vi "pco.labview_LightSheet_Example.vi"() -> ()   [LabVIEW 2019]
uses:
  pco.sdk/CameraAccess/CameraAccess.lvlib
  pco.sdk/Structures/Structures.lvlib
  pco.recorder/Recorder.lvlib
  pco.sdk/RecordingControl/RecordingControl.lvlib
  pco.sdk/TimingControl/TimingControl.lvlib
  pco.sdk/GeneralCameraControl/GeneralCameraControl.lvlib
  pco.sdk/SpecialCommandsEdge/SpecialCommandsEdge.lvlib
panel:
  in  "dwExposureLines":u32=100
  in  "wTimeBase":u16(ring)=1 items=["ns", "us", "ms"]
  in  "dwLineTime":u32=50
  out "Recorded Images":u32
  out "Image":u16[][](graph)
  in  "Quit":bool
  in  "roiY1":u16=2 min=2 step=1
  in  "roiX1":u16=2 min=2 step=1
  in  "roiY0":u16=1 min=1 step=1
  in  "roiX0":u16=1 min=1 step=1
  out "Image Height":u16
  out "Image Width":u16
  in  "Image Index":u32 max=9
  in  "dwImgCount":u32=10 caption="Required Number of Images" max=4023
  out "Error":errorcluster {"code" format="%x"}
  # "This example is similar to the simple example, but uses get/set line timeing for controlling the exposure.\nExposureTime = LineTime * ExposureLines\nBeside of the line timing part, a simple recording of an image sequence and the image access afterwards is done.\nIt is a good starting point for writing own applications, especially  for light sheet application development.\nBut it will not be fail save, i.e. doesnt react on errors, just handles them forward to the end\n\nUsage:\nSelect your required image count and the required line tiime + number of exposure lines before you start the program.\nOnce started, the camera will be opened, the recorder will be created, initialized and images will be recorded automatically.\nWhen acquisition has finished you can address the images and set a certain roi \nTo finish the program click on quit application, this will force free and delete of the recorder and a close camera"
  # "pco.labview"
  # "Camera Setup"
  # "Recording Control"
  # "Parameters for image readout"
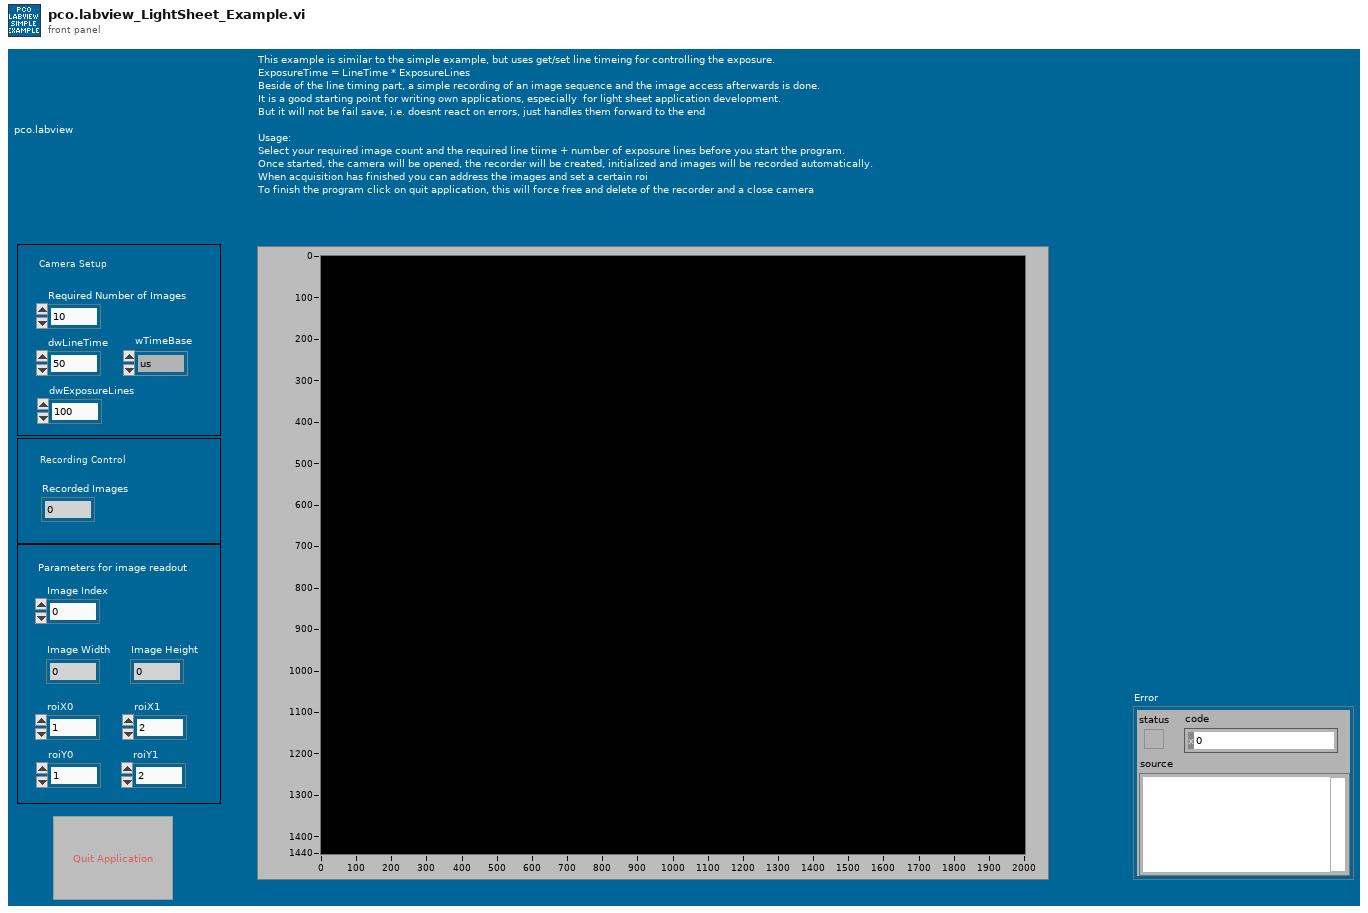
[diagram p1: front panel]
types:
  T1 = enum8{"Enabled", "Disabled", "Disabled and Grayed Out"}
  T2 = cluster{"wInterfaceType":u16, "wCameraNumber":u16, "wCameraNumAtInterface":u16, "wOpenFlags":u16[], "dwOpenFlags":u32[], "wOpenPtr":u64[]}
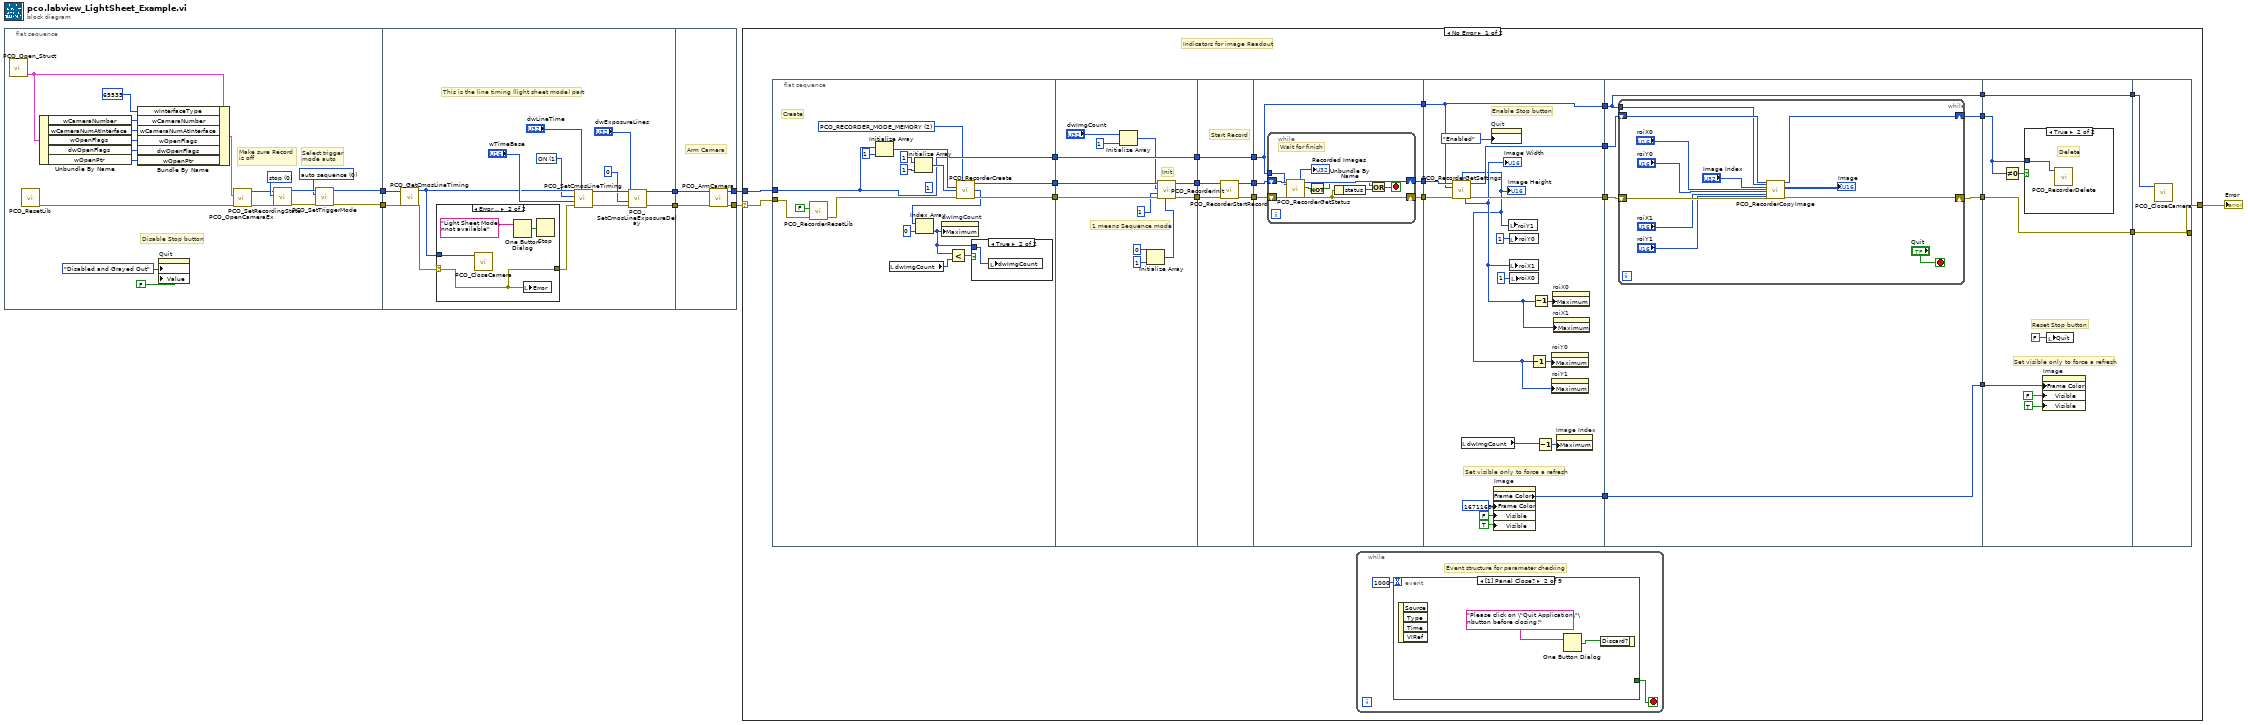
[diagram p0: block diagram]
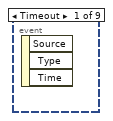
[diagram p3: hidden frame]
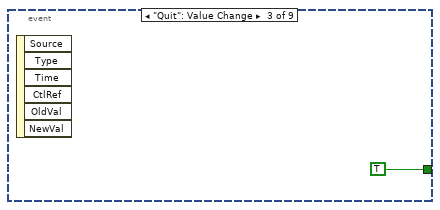
[diagram p4: hidden frame]
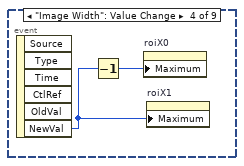
[diagram p5: hidden frame]
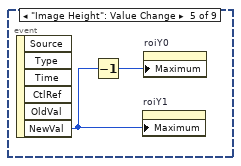
[diagram p6: hidden frame]
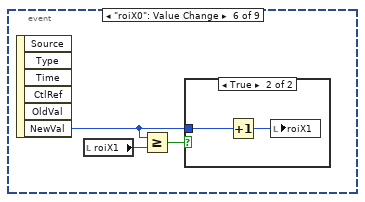
[diagram p7: hidden frame]
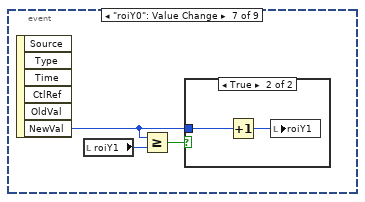
[diagram p9: hidden frame]
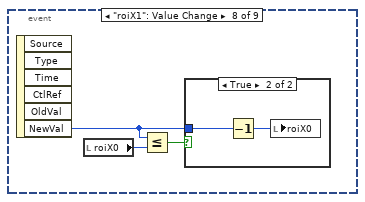
[diagram p11: hidden frame]
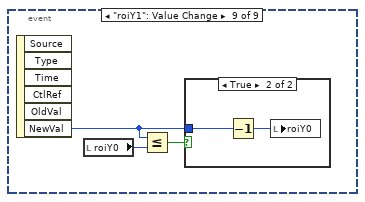
[diagram p13: hidden frame]
diagram:
  n1 = flat-sequence {
    tunnel: [w9] -> w4
    tunnel: [w8] -> w3
    tunnel: w4 -> [w39]
    tunnel: w3 -> [w40]
    tunnel: [w30] -> w2
    tunnel: [w29] -> w1
    tunnel: [w48] -> w5
    tunnel: [w49] -> w7
    tunnel: w2 -> [w47]
    tunnel: w1 -> [w46]
    frame #0 {
      w10 = u16 0 items=["auto sequence"=0, "software trigger"=1, "external exposure start & software trigger"=2, "external exposure control"=3, "external synchronized"=4, "fast external exposure control"=5, "external CDS control"=6, "slow external exposure control"=7, "external synchronized HDSDI"=258] ("wTriggerMode")
      w15 = u16 0 items=["stop", "run"] ("wRecState")
      # "Select trigger\nmode auto"
      # "Make sure Record \nis off"
      # "Disable Stop button"
      n2 = call "PCO_Open_Struct.vi"() -> ("PCO_Open_Struct"=w22:T2)  [unwired: 4 in, 4 out]
      n3 = call "PCO_ResetLib.vi"() -> ("error out"=w26:errorcluster)  [unwired: 10 in, 1 out]
      n4 = Unbundle By Name(w22) -> ("wCameraNumber"=w21:u16, "wCameraNumAtInterface"=w20:u16, "wOpenFlags"=w19:u16[], "dwOpenFlags"=w18:u32[], "wOpenPtr"=w17:u64[])
      n5 = Bundle By Name(cluster=w22, "wInterfaceType"=u16 65535, "wCameraNumber"=w21, "wCameraNumAtInterface"=w20, "wOpenFlags"=w19, "dwOpenFlags"=w18, "wOpenPtr"=w17) -> (w16:T2)
      n6 = property on="Quit" class="Bool (strict)"("DisabledEnum"=T1."Disabled and Grayed Out" ("Disabled"), "Value"=FALSE ("Stop")) -> ()  [unwired: 2 in, 2 out]
      n7 = call "PCO_OpenCameraEx.vi"("error in (no error)"=w26, "strOpenStruct"=w16) -> ("error out"=w14:errorcluster, "ph out"=w13:u64)  [unwired: 7 in, 1 out]
      n8 = call "PCO_SetRecordingState.vi"("error in (no error)"=w14, "wRecState"=w15, "ph"=w13) -> ("error out"=w11:errorcluster, "ph out"=w12:u64)  [unwired: 6 in, 1 out]
      n9 = call "PCO_SetTriggerMode.vi"("error in (no error)"=w11, "wTriggerMode"=w10, "ph"=w12) -> ("error out"=w8:errorcluster, "ph out"=w9:u64)  [unwired: 6 in, 1 out]
    }
    frame #1 {
      w27 = u16 1 items=["OFF", "ON"] ("wParameter")
      # "This is the line timing (light sheet mode) part"
      n10 = call "PCO_GetCmosLineTiming.vi"("ph"=w39, "error in (no error)"=w40) -> ("ph out"=w28:u64, "error out"=w38:errorcluster)  [unwired: 10 in, 6 out]
      n11 = case shown="Error .." w38 {
        selector: w38 -> [w41 w42]
        tunnel: [w41 w42] -> w37
        tunnel: w28 -> [_ w43]
        frame No Error {
        }
        frame Error {
          n12 = call "PCO_CloseCamera.vi"("ph"=w43) -> ()  [unwired: 9 in, 2 out]
          n13 = One Button Dialog(message="Light Sheet Mode\nnot available") -> (true=w44:bool)  [unwired: 1 in]
          n14 = local write "Error"(w42) -> ()
          n15 = Stop(stop? (T)=w44) -> ()
        }
      }
      n16 = call "PCO_SetCmosLineTiming.vi"("dwLineTime"="dwLineTime", "error in (no error)"=w37, "wTimeBase"="wTimeBase", "wParameter"=w27, "ph"=w28) -> ("error out"=w33:errorcluster, "ph out"=w34:u64)  [unwired: 4 in, 1 out]
      n17 = call "PCO_SetCmosLineExposureDelay.vi"("error in (no error)"=w33, "dwDelayLines"=u32 0, "dwExposureLines"="dwExposureLines", "ph"=w34) -> ("error out"=w29:errorcluster, "ph out"=w30:u64)  [unwired: 5 in, 1 out]
    }
    frame #2 {
      # "Arm Camera"
      n18 = call "PCO_ArmCamera.vi"("error in (no error)"=w46, "ph"=w47) -> ("error out"=w48:errorcluster, "ph out"=w49:u64)  [unwired: 7 in, 1 out]
    }
  }
  n19 = case shown="No Error" w5 {
    selector: w5 -> [w54 w201]
    tunnel: [w50 w201] -> w6
    tunnel: w7 -> [w74 _]
    frame No Error {
      # "Indicators for image Readout"
      n20 = flat-sequence {
        tunnel: w74 -> [w114]
        tunnel: w54 -> [w111]
        tunnel: [w113] -> w73
        tunnel: [w115] -> w72
        tunnel: [w114] -> w61
        tunnel: w73 -> [w133]
        tunnel: w72 -> [w129]
        tunnel: [w132] -> w71
        tunnel: [w131] -> w70
        tunnel: [w130] -> w62
        tunnel: w61 -> [w130]
        tunnel: w71 -> [w138]
        tunnel: w70 -> [w137]
        tunnel: [w136] -> w69
        tunnel: [w135] -> w68
        tunnel: [w134] -> w63
        tunnel: w62 -> [w134]
        tunnel: w69 -> [w143]
        tunnel: w68 -> [w142]
        tunnel: [w141] -> w67
        tunnel: [w140] -> w66
        tunnel: w63 -> [w139]
        tunnel: [w139] -> w60
        tunnel: w67 -> [w170]
        tunnel: w66 -> [w169]
        tunnel: [w168] -> w65
        tunnel: [w167] -> w64
        tunnel: w60 -> [w166]
        tunnel: [w166] -> w59
        tunnel: [w162] -> w53
        tunnel: w65 -> [w177]
        tunnel: w64 -> [w176]
        tunnel: w59 -> [w173]
        tunnel: [w175] -> w58
        tunnel: [w174] -> w57
        tunnel: [w173] -> w56
        tunnel: w53 -> [w172]
        tunnel: [w172] -> w52
        tunnel: w58 -> [w190]
        tunnel: w57 -> [w196]
        tunnel: w56 -> [w194]
        tunnel: [w194] -> w55
        tunnel: w52 -> [w191]
        tunnel: [w190] -> w51
        tunnel: w55 -> [w200]
        tunnel: w51 -> [w199]
        tunnel: [w199] -> w50
        frame #0 {
          w104 = u16 2 items=["PCO_RECORDER_MODE_FILE"=1, "PCO_RECORDER_MODE_MEMORY"=2, "PCO_RECORDER_MODE_CAMRAM"=3] ("dwRecMode")
          (unwired) u16 1 ("wArrLength")
          # "Create"
          n21 = call "PCO_RecorderResetLib.vi"("error in (no error)"=w111, "bSilent"=FALSE) -> ("error out"=w110:errorcluster)  [unwired: 8 in, 1 out]
          n22 = Initialize Array(w114, u32 1 ("element")) -> (w119:u64[])
          n23 = local read "dwImgCount"() -> (w107:u32)
          n24 = Initialize Array(u32 1 ("element"), u32 1 ("element")) -> (w116:u32[])
          n25 = call "PCO_RecorderCreate.vi"("wRecMode"=w104, "phCamArr"=w119, "dwImgDistributionArr"=w116, "error in (no error)"=w110) -> ("phRec out"=w113:u64, "dwMaxImgCountArr"=w109:u32[], "error out"=w115:errorcluster)  [unwired: 8 in, 1 out]
          n26 = Index Array(array=w109, index=0) -> (element=w106:u32)
          n27 = property on="dwImgCount" class="DigNum (strict)"("Maximum"=w106) -> ()  [unwired: 2 in, 2 out]
          n28 = Less?(x=w106, y=w107) -> (x < y?=w105:bool)
          n29 = case shown="True" w105 {
            tunnel: w106 -> [_ w121]
            frame False {
            }
            frame True {
              n30 = local write "dwImgCount"(w121) -> ()
            }
          }
        }
        frame #1 {
          # "1 means Sequence mode"
          # "Init"
          n31 = Initialize Array("dwImgCount", 1 ("dimension size")) -> (w126:u32[])
          n32 = Initialize Array(u16 0 ("element"), 1 ("dimension size")) -> (w122:u16[])
          n33 = call "PCO_RecorderInit.vi"("wRamSegmentArr"=w122, "error in (no error)"=w129, "wType"=u16 1, "dwImgCountArr"=w126, "phRec"=w133) -> ("error out"=w131:errorcluster, "phRec out"=w132:u64)  [unwired: 4 in, 1 out]
        }
        frame #2 {
          # "Start Record"
          n34 = call "PCO_RecorderStartRecord.vi"("error in (no error)"=w137, "phRec"=w138) -> ("error out"=w136:errorcluster, "phRec out"=w135:u64)  [unwired: 7 in, 1 out]
        }
        frame #3 {
          n35 = while {
            shift-right: [w152] -> w140
            shift-left: w143 -> [w153]
            shift-right: [w148] -> w141
            shift-left: w142 -> [w149]
            tunnel: w139 -> [w147]
            stop <- w150 stop-if-true
            # "Wait for finish"
            n36 = call "PCO_RecorderGetStatus.vi"("phRec"=w149, "phCam"=w147, "error in (no error)"=w153) -> ("dwProcImgCount"=→"Recorded Images":u32, "phRec out"=w148:u64, "bIsRunning"=w146:bool, "error out"=w152:errorcluster)  [unwired: 5 in, 8 out]
            n37 = Not(x=w146) -> (.not. x?=w145:bool)
            n38 = Unbundle By Name(w152) -> ("status"=w151:bool)
            n39 = Or(x=w145, y=w151) -> (x .or. y?=w150:bool)
          }
        }
        frame #4 {
          # "Set visible only to force a refresh"
          # "Enable Stop button"
          n40 = call "PCO_RecorderGetSettings.vi"("phRec"=w170, "phCam"=w166, "error in (no error)"=w169) -> ("wHeight"=w155:u16, "phRec out"=w168:u64, "wWidth"=w156:u16, "error out"=w167:errorcluster)  [unwired: 4 in, 5 out]
          "Image Width" <- w156
          "Image Height" <- w155
          n41 = local read "dwImgCount"() -> (w154:u32)
          n42 = property on="Quit" class="Bool (strict)"("DisabledEnum"=T1."Enabled" ("Disabled")) -> ()  [unwired: 2 in, 2 out]
          n43 = property on="Image" class="IntGraph (strict)"("Frame Color"=u32 16711680, "Visible"=FALSE, "Visible"=TRUE) -> ("Frame Color"=w162:u32)  [unwired: 2 in, 2 out]
          n44 = local write "roiY1"(w155) -> ()
          n45 = local write "roiY0"(u16 1 ("roiY0")) -> ()
          n46 = local write "roiX1"(w156) -> ()
          n47 = local write "roiX0"(u16 1 ("roiY0")) -> ()
          n48 = Decrement(x=w155) -> (x-1=w158:u16)
          n49 = Decrement(x=w156) -> (x-1=w159:u16)
          n50 = Decrement(x=w154) -> (x-1=w157:u32)
          n51 = property on="roiY0" class="DigNum (strict)"("Maximum"=w158) -> ()  [unwired: 2 in, 2 out]
          n52 = property on="roiY1" class="DigNum (strict)"("Maximum"=w155) -> ()  [unwired: 2 in, 2 out]
          n53 = property on="roiX0" class="DigNum (strict)"("Maximum"=w159) -> ()  [unwired: 2 in, 2 out]
          n54 = property on="roiX1" class="DigNum (strict)"("Maximum"=w156) -> ()  [unwired: 2 in, 2 out]
          n55 = property on="Image Index" class="DigNum (strict)"("Maximum"=w157) -> ()  [unwired: 2 in, 2 out]
        }
        frame #5 {
          n56 = while {
            tunnel: w173 -> [w186]
            shift-right: [w185] -> w174
            shift-left: w177 -> [w188]
            shift-right: [w184] -> w175
            shift-left: w176 -> [w187]
            stop <- "Quit" stop-if-true
            n57 = call "PCO_RecorderCopyImage.vi"("phRec"=w188, "phCam"=w186, "dwImgIdx"="Image Index", "wRoiX0"="roiX0", "wRoiY0"="roiY0", "wRoiX1"="roiX1", "wRoiY1"="roiY1", "error in (no error)"=w187) -> ("phRec out"=w185:u64, "wImgBuf"=→"Image":u16[][], "error out"=w184:errorcluster)  [unwired: 13 in, 4 out]
          }
        }
        frame #6 {
          # "Set visible only to force a refresh"
          # "Reset Stop button"
          n58 = Not Equal To 0?(x=w196) -> (x != 0?=w195:bool)
          n59 = case shown="True" w195 {
            tunnel: w196 -> [_ w198]
            frame False {
            }
            frame True {
              # "Delete"
              n60 = call "PCO_RecorderDelete.vi"("phRec"=w198) -> ()  [unwired: 9 in, 2 out]
            }
          }
          n61 = property on="Image" class="IntGraph (strict)"("Frame Color"=w191, "Visible"=FALSE, "Visible"=TRUE) -> ()  [unwired: 2 in, 2 out]
          n62 = local write "Quit"(FALSE ("Stop")) -> ()
        }
        frame #7 {
          n63 = call "PCO_CloseCamera.vi"("ph"=w200) -> ()  [unwired: 9 in, 2 out]
        }
      }
      n64 = while {
        stop <- w75 stop-if-true
        # "Event structure for parameter checking"
        n65 = event shown="[1] Panel Close?" {
          selector: _ -> [_ _ _ _ _ _ _ _ _]
          dyn-events: _ -> [_ _ _ _ _ _ _ _ _]
          timeout: 1000 -> [_ _ _ _ _ _ _ _ _]
          tunnel: [_ _ TRUE _ _ _ _ _ _] -> w75
          event Timeout {
            n66 = event-data() -> ()  [unwired: 1 in, 3 out]
          }
          event Panel Close? {
            n67 = event-data() -> ()  [unwired: 1 in, 4 out]
            n68 = One Button Dialog(message="Please click on \"Quit Application\"\nbutton before closing!") -> (true=w77:bool)  [unwired: 1 in]
            n69 = event-data("Discard?"=w77) -> ()  [unwired: 1 in, 1 out]
          }
          event "Quit": Value Change {
            n70 = event-data() -> ()  [unwired: 1 in, 6 out]
          }
          event "Image Width": Value Change {
            n71 = event-data() -> ("NewVal"=w80:u16)  [unwired: 1 in, 5 out]
            n72 = Decrement(x=w80) -> (x-1=w81:u16)
            n73 = property on="roiX0" class="DigNum (strict)"("Maximum"=w81) -> ()  [unwired: 2 in, 2 out]
            n74 = property on="roiX1" class="DigNum (strict)"("Maximum"=w80) -> ()  [unwired: 2 in, 2 out]
          }
          event "Image Height": Value Change {
            n75 = event-data() -> ("NewVal"=w82:u16)  [unwired: 1 in, 5 out]
            n76 = Decrement(x=w82) -> (x-1=w83:u16)
            n77 = property on="roiY1" class="DigNum (strict)"("Maximum"=w82) -> ()  [unwired: 2 in, 2 out]
            n78 = property on="roiY0" class="DigNum (strict)"("Maximum"=w83) -> ()  [unwired: 2 in, 2 out]
          }
          event "roiX0": Value Change {
            n79 = event-data() -> ("NewVal"=w84:u16)  [unwired: 1 in, 5 out]
            n80 = local read "roiX1"() -> (w86:u16)
            n81 = Greater Or Equal?(x=w84, y=w86) -> (x >= y?=w85:bool)
            n82 = case shown="True" w85 {
              tunnel: w84 -> [_ w88]
              frame False {
              }
              frame True {
                n83 = Increment(x=w88) -> (x+1=w87:u16)
                n84 = local write "roiX1"(w87) -> ()
              }
            }
          }
          event "roiY0": Value Change {
            n85 = event-data() -> ("NewVal"=w89:u16)  [unwired: 1 in, 5 out]
            n86 = local read "roiY1"() -> (w91:u16)
            n87 = Greater Or Equal?(x=w89, y=w91) -> (x >= y?=w90:bool)
            n88 = case shown="True" w90 {
              tunnel: w89 -> [_ w93]
              frame False {
              }
              frame True {
                n89 = Increment(x=w93) -> (x+1=w92:u16)
                n90 = local write "roiY1"(w92) -> ()
              }
            }
          }
          event "roiX1": Value Change {
            n91 = event-data() -> ("NewVal"=w94:u16)  [unwired: 1 in, 5 out]
            n92 = local read "roiX0"() -> (w96:u16)
            n93 = Less Or Equal?(x=w94, y=w96) -> (x <= y?=w95:bool)
            n94 = case shown="True" w95 {
              tunnel: w94 -> [_ w98]
              frame False {
              }
              frame True {
                n95 = Decrement(x=w98) -> (x-1=w97:u16)
                n96 = local write "roiX0"(w97) -> ()
              }
            }
          }
          event "roiY1": Value Change {
            n97 = event-data() -> ("NewVal"=w99:u16)  [unwired: 1 in, 5 out]
            n98 = local read "roiY0"() -> (w101:u16)
            n99 = Less Or Equal?(x=w99, y=w101) -> (x <= y?=w100:bool)
            n100 = case shown="True" w100 {
              tunnel: w99 -> [_ w103]
              frame False {
              }
              frame True {
                n101 = Decrement(x=w103) -> (x-1=w102:u16)
                n102 = local write "roiY0"(w102) -> ()
              }
            }
          }
        }
      }
    }
    frame Error {
    }
  }
  "Error" <- w6
